vi "Carica misure.vi"(6 "Filtro 3ph6ch":bool[](array[boolean]), 8 "error in (no error)":errorcluster, 10 "ID bollettino":string[](array[string]), 11 "Refnum in":T2) -> (0 "error out":errorcluster, 2 "Dati prove out":T1, 3 "Refnum out":T2)   [LabVIEW 2019]
uses:
  <vilib>/addons/database/Connection.llb/Conn ObjectReference.ctl
  TypeDef/Dati collaudo.ctl
  <vilib>/addons/database/_DB Variant To Data/Database Variant To Data.xnode
  <vilib>/addons/database/NI_Database_API.lvlib
panel:
  out "data":string[][][](array[string])
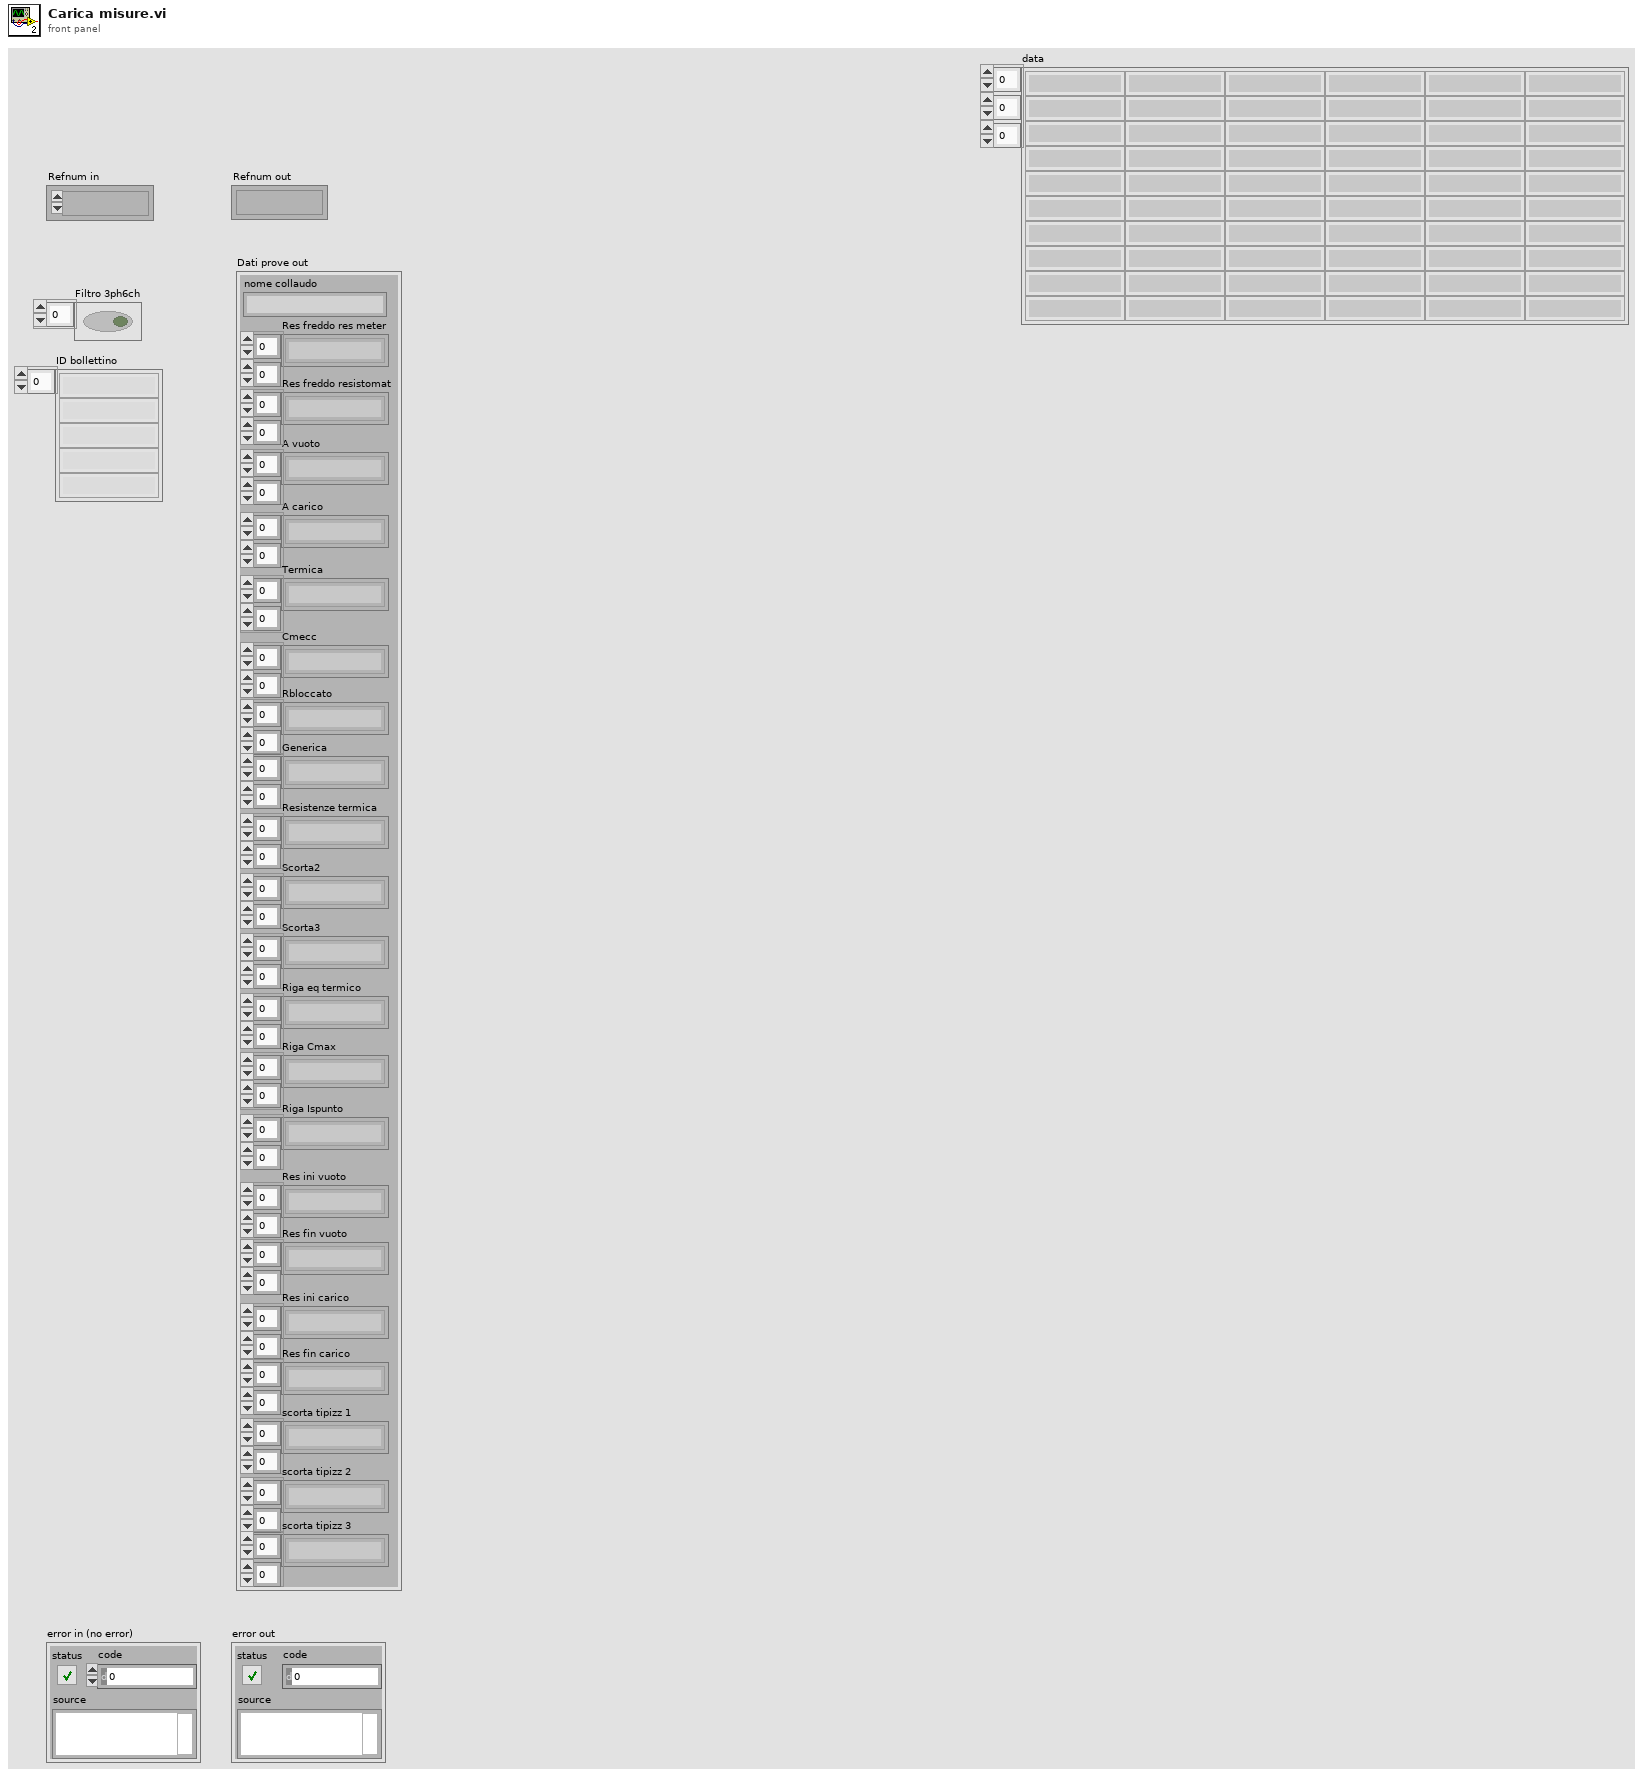
[diagram p1: front panel]
types:
  T1 = typedef "Dati collaudo.ctl" = cluster{"nome collaudo":string, "Res freddo res meter":string[][], "Res freddo resistomat":string[][], "A vuoto":string[][], "A carico":string[][], "Termica":string[][], "Cmecc":string[][], "Rbloccato":string[][], "Generica":string[][], "Resistenze termica":string[][], "Scorta2":string[][], "Scorta3":string[][], "Riga eq termico":string[][], "Riga Cmax":string[][], "Riga Ispunto":string[][], "Res ini vuoto":string[][], "Res fin vuoto":string[][], "Res ini carico":string[][], "Res fin carico":string[][], "scorta tipizz 1":string[][], "scorta tipizz 2":string[][], "scorta tipizz 3":string[][]}
  T2 = typedef "NI_Database_API.lvlib/Conn ObjectReference.ctl" = refnum<k1>
  T3 = cluster{"BANCO":string, "ANNO":string, "PROGRESSIVO":string, "TIPO PROVA":string, "PROVA SPECIALE ?":string, "DATA":string}
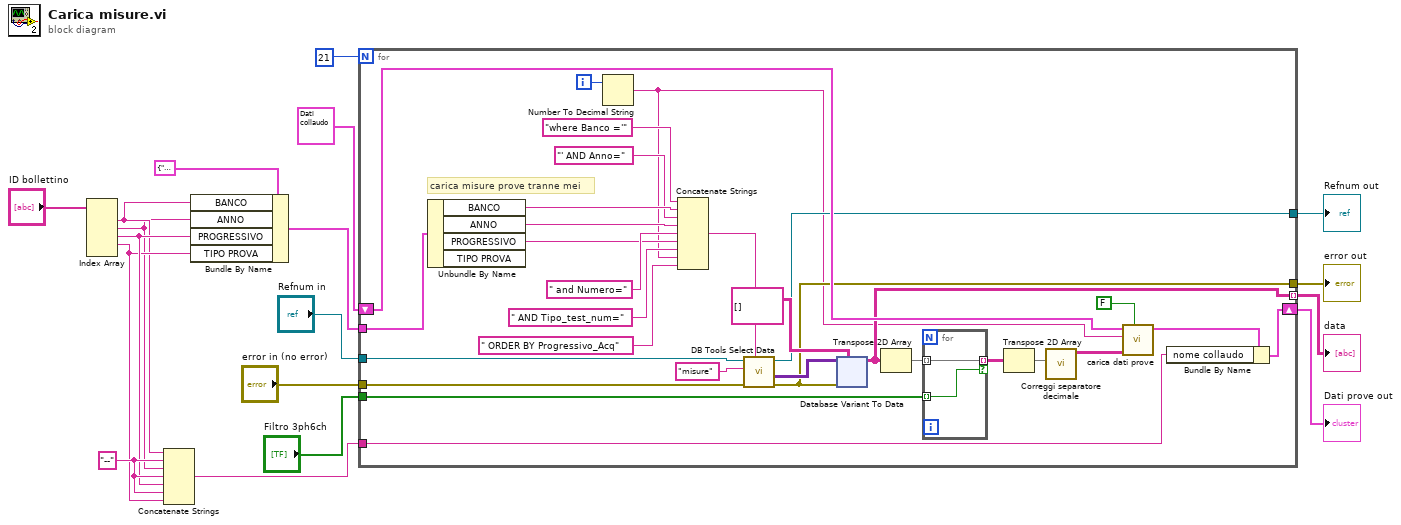
[diagram p0: block diagram]
diagram:
  w7 = "--" ("string")
  n1 = Index Array(array="ID bollettino") -> (element #1=w3:string, element #2=w2:string, element #3=w5:string, element #4=w4:string)  [unwired: 5 in, 1 out]
  n2 = Concatenate Strings(w3, w7, w2, w7, w5, w7, w4) -> (w6:string)
  n3 = Bundle By Name(cluster=T3 {"BANCO"="0", "ANNO"="17", "PROGRESSIVO"="12", "TIPO PROVA"="F", "PROVA SPECIALE ?"="NO", "DATA"="29/11/2017 10:25:21"} ("bollettino"), "BANCO"=w3, "ANNO"=w2, "PROGRESSIVO"=w5, "TIPO PROVA"=w4) -> (w18:T3)
  n4 = for {
    N: 21 -> [_]
    tunnel: "Refnum in" -> [w46]
    tunnel: "error in (no error)" -> [w45]
    shift-right: [w40] -> w11
    shift-left: T1 {"nome collaudo"="", "Res freddo res meter"=[], "Res freddo resistomat"=[], "A vuoto"=[], "A carico"=[], "Termica"=[], "Cmecc"=[], "Rbloccato"=[], "Generica"=[], "Resistenze termica"=[], "Scorta2"=[], "Scorta3"=[], "Riga eq termico"=[], "Riga Cmax"=[], "Riga Ispunto"=[], "Res ini vuoto"=[], "Res fin vuoto"=[], "Res ini carico"=[], "Res fin carico"=[], "scorta tipizz 1"=[], "scorta tipizz 2"=[], "scorta tipizz 3"=[]} ("Dati prove out") -> [w42]
    tunnel: w18 -> [w34]
    tunnel: [w33] -> w13
    tunnel: [w32] -> w14
    tunnel: "Filtro 3ph6ch" -> [w27]
    tunnel: w6 -> [w26]
    tunnel: [w21] -> w1 mode=indexing
    i -> [w39]
    # "carica misure prove tranne mei"
    n5 = Unbundle By Name(w34) -> ("BANCO"=w24:string, "ANNO"=w22:string, "PROGRESSIVO"=w36:string)  [unwired: 1 out]
    n6 = Number To Decimal String(number=w39) -> (decimal integer string=w20:string)  [unwired: 1 in]
    n7 = Concatenate Strings("where Banco ='" ("string"), w24, "' AND Anno=" ("string"), w22, " and Numero=" ("string"), w36, " AND Tipo_test_num=" ("string"), w20, " ORDER BY Progressivo_Acq" ("string")) -> (w44:string)
    n8 = call <vilib>:"DB Tools Select Data.vi"("condition"=w44, "error in (no error)"=w45, "table"="misure", "connection reference"=w46) -> ("error out"=w32:errorcluster, "data"=w48:variant[][], "connection reference out"=w33:T2)  [unwired: 2 in]
    n9 = xnode "Database Variant To Data"("database variant"=w48, "error in (no error)"=w32, "type"=string[][] []) -> ("data"=w21:string[][])  [unwired: 1 out]
    n10 = Transpose 2D Array(2D array=w21) -> (transposed array=w29:string[][])
    n11 = for {
      tunnel: w27 -> [w49] mode=indexing
      tunnel: w29 -> [w50] mode=indexing
      tunnel: [w50] -> w30 mode=indexing if=w49
    }
    n12 = Transpose 2D Array(2D array=w30) -> (transposed array=w28:string[][])
    n13 = call "Correggi separatore decimale.vi"("Array in"=w28) -> ("Array out"=w31:string[][])  [unwired: 10 in]
    n14 = call "carica dati prove.vi"("Carica tabelle?"=FALSE, "Dati in"=w31, "prova"=w20, "Dati prove in"=w42) -> ("Dati prove out"=w41:T1)  [unwired: 5 in, 2 out]
    n15 = Bundle By Name(cluster=w41, "nome collaudo"=w26) -> (w40:T1)
  }
  "error out" <- w14
  "Refnum out" <- w13
  "Dati prove out" <- w11
  "data" <- w1
